vi "Configure Marker Type.vi"(0 "VISA resource name":refnum<visa-resource-name>, 1 "X (0 Hz)":dbl, 2 "Center X (0)":dbl, 3 "X Span (0)":dbl, 5 "Active Marker (1: Marker1)":u16(ring)=1 items=["Marker1"=1, "Marker2"=2, "Marker3"=3, "Marker4"=4], 7 "Marker Type (1: Position)":u16(ring)=1 items=["Off", "Position", "Delta", "Band", "Span Pair"], 9 "Readout (0: Frequency)":u16(ring) items=["Frequency", "Time", "Inverse Time", "Period"], 11 "error in (no error)":errorcluster, 12 "X Start (0)":dbl, 13 "X Stop (0)":dbl) -> (4 "VISA resource name out":refnum<visa-resource-name>, 15 "error out":errorcluster)   [LabVIEW 2014, in "Agilent ESA PSA Series.lvlib"]
doc: "Configures the marker type settings of the selected marker."
uses:
  Agilent ESA PSA Series.lvlib
panel:
  # "Span Pair"
  # "Band"
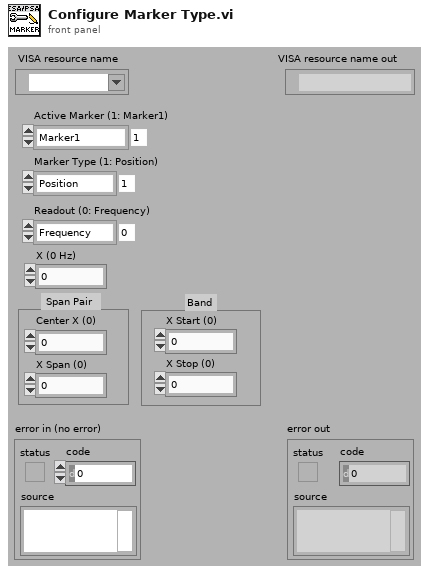
[diagram p1: front panel]
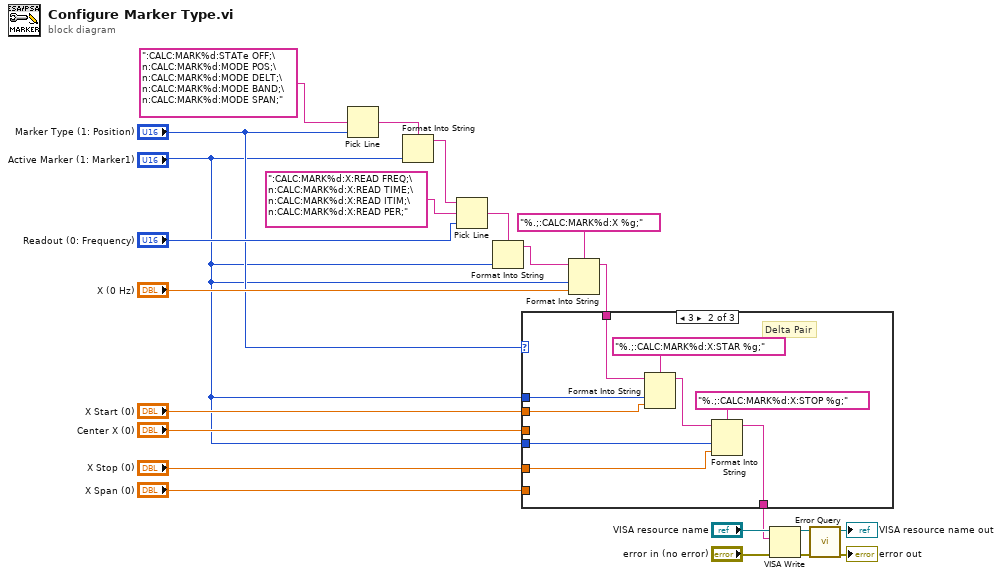
[diagram p0: block diagram]
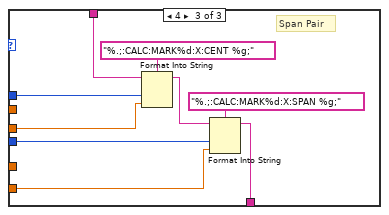
[diagram p3: hidden frame]
diagram:
  n1 = Pick Line(multi-line string=":CALC:MARK%d:STATe OFF;\n:CALC:MARK%d:MODE POS;\n:CALC:MARK%d:MODE DELT;\n:CALC:MARK%d:MODE BAND;\n:CALC:MARK%d:MODE SPAN;", line index="Marker Type (1: Position)") -> (output string=w16:string)  [unwired: 1 in]
  n2 = Format Into String(format string=w16, "Active Marker (1: Marker1)") -> (resulting string=w13:string)  [unwired: 2 in, 1 out]
  n3 = Pick Line(string ("")=w13, multi-line string=":CALC:MARK%d:X:READ FREQ;\n:CALC:MARK%d:X:READ TIME;\n:CALC:MARK%d:X:READ ITIM;\n:CALC:MARK%d:X:READ PER;", line index="Readout (0: Frequency)") -> (output string=w12:string)
  n4 = Format Into String(format string=w12, "Active Marker (1: Marker1)") -> (resulting string=w10:string)  [unwired: 2 in, 1 out]
  n5 = Format Into String(format string="%.;:CALC:MARK%d:X %g;", initial string=w10, "Active Marker (1: Marker1)", "X (0 Hz)") -> (resulting string=w7:string)  [unwired: 1 in, 1 out]
  n6 = case shown="3" "Marker Type (1: Position)" {
    tunnel: "Active Marker (1: Marker1)" -> [_ w30 w38]
    tunnel: "Active Marker (1: Marker1)" -> [_ w29 w37]
    tunnel: w7 -> [w24 w28 w39]
    tunnel: [w24 w27 w36] -> w6
    tunnel: "X Start (0)" -> [_ w26 _]
    tunnel: "X Stop (0)" -> [_ w25 _]
    tunnel: "Center X (0)" -> [_ _ w35]
    tunnel: "X Span (0)" -> [_ _ w34]
    frame 0, Default {
    }
    frame 3 {
      # "Delta Pair"
      n7 = Format Into String(format string="%.;:CALC:MARK%d:X:STAR %g;", initial string=w28, w30, w26) -> (resulting string=w33:string)  [unwired: 1 in, 1 out]
      n8 = Format Into String(format string="%.;:CALC:MARK%d:X:STOP %g;", initial string=w33, w29, w25) -> (resulting string=w27:string)  [unwired: 1 in, 1 out]
    }
    frame 4 {
      # "Span Pair"
      n9 = Format Into String(format string="%.;:CALC:MARK%d:X:CENT %g;", initial string=w39, w38, w35) -> (resulting string=w42:string)  [unwired: 1 in, 1 out]
      n10 = Format Into String(format string="%.;:CALC:MARK%d:X:SPAN %g;", initial string=w42, w37, w34) -> (resulting string=w36:string)  [unwired: 1 in, 1 out]
    }
  }
  n11 = VISA Write(VISA resource name="VISA resource name", write buffer=w6, error in (no error)="error in (no error)") -> (VISA resource name out=w21:refnum<visa-resource-name>, error out=w19:errorcluster)  [unwired: 1 out]
  n12 = call "Error Query.vi"("error in (no error)"=w19, "VISA resource name"=w21) -> ("error out"=→"error out":errorcluster, "VISA resource name out"=→"VISA resource name out":refnum<visa-resource-name>)  [unwired: 6 in, 2 out]
